vi "Buffer.vi"(4 "Error In":errorcluster, 5 "Plugin Names":T1, 6 "Function":enum16{"Read", "Insert"}(ring), 7 "VI Ref In":refnum<vi>) -> (0 "Error Out":errorcluster, 3 "VI Ref Out":refnum<vi>)   [LabVIEW 2015, in "Plugin References.lvlib"]
uses:
  Plugin References.lvlib
  _libraries/Startup Processes/_typedefs/Subpanel Names.ctl
  _libraries/Startup Processes/Startup Processes.lvlib
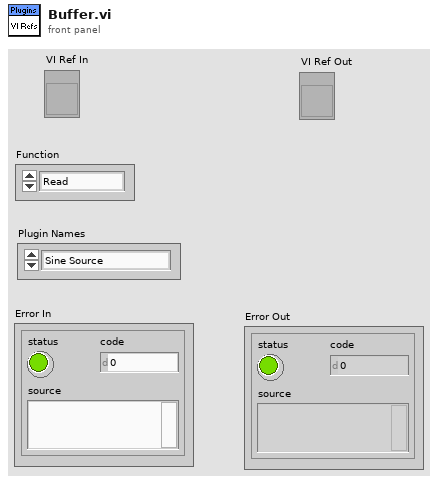
[diagram p1: front panel]
types:
  T1 = typedef "Startup Processes.lvlib/Subpanel Names.ctl" = enum16{"Sine Source", "Ramp Source", "Hen House TC", "Dog House TC", "Out House TC"}
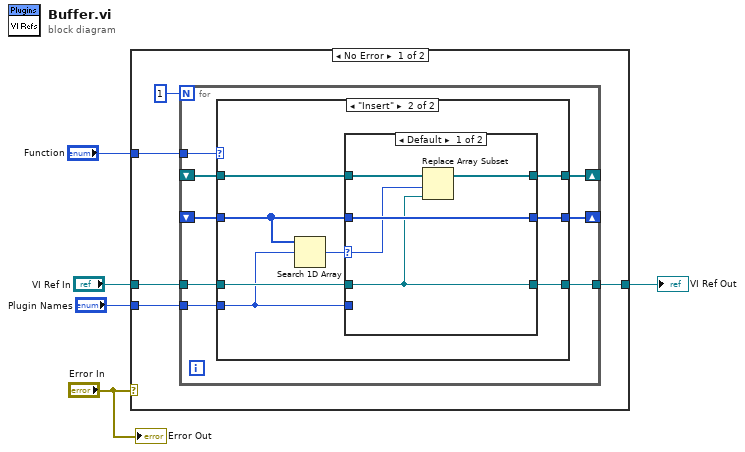
[diagram p0: block diagram]
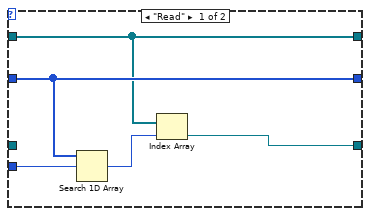
[diagram p2: hidden frame]
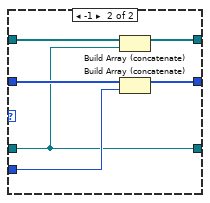
[diagram p3: hidden frame]
diagram:
  n1 = case shown="No Error" "Error In" {
    tunnel: "Function" -> [w9 _]
    tunnel: "VI Ref In" -> [w8 _]
    tunnel: "Plugin Names" -> [w7 _]
    tunnel: [w6 _] -> w1
    frame No Error {
      n2 = for {
        N: 1 -> [_]
        tunnel: w9 -> [w18]
        shift-right: [w16] -> _
        shift-left: _ -> [w17]
        tunnel: w8 -> [w15]
        shift-right: [w14] -> _
        shift-left: _ -> [w13]
        tunnel: w7 -> [w12]
        tunnel: [w11] -> w6
        n3 = case shown="\"Insert\"" w18 {
          tunnel: w17 -> [w22 w26]
          tunnel: [w22 w31] -> w16
          tunnel: w15 -> [_ w28]
          tunnel: w13 -> [w21 w29]
          tunnel: [w21 w30] -> w14
          tunnel: w12 -> [w23 w27]
          tunnel: [w19 w24] -> w11
          frame "Read" {
            n4 = Search 1D Array(1D array=w22, element=w23) -> (index of element=w20:i32)  [unwired: 1 in]
            n5 = Index Array(array=w21, index=w20) -> (element=w19:refnum<vi>)
          }
          frame "Insert" {
            n6 = Search 1D Array(1D array=w26, element=w27) -> (index of element=w25:i32)  [unwired: 1 in]
            n7 = case shown="Default" w25 {
              selector: w25 -> [w33 _]
              tunnel: [w36 w42] -> w31
              tunnel: [w34 w41] -> w30
              tunnel: w29 -> [w35 w40]
              tunnel: w28 -> [w32 w37]
              tunnel: w27 -> [_ w39]
              tunnel: w26 -> [w36 w38]
              tunnel: [w32 w37] -> w24
              frame Default {
                n8 = Replace Array Subset(array=w35, new element=w32, index=w33) -> (w34:refnum<vi>[])
              }
              frame -1 {
                n9 = Build Array (concatenate)(w40, w37) -> (w41:refnum<vi>[])
                n10 = Build Array (concatenate)(w38, w39) -> (w42:T1[])
              }
            }
          }
        }
      }
    }
    frame Error {
    }
  }
  "VI Ref Out" <- w1
  "Error Out" <- "Error In"
